vi "Loader RT Post-Build Action.vi"(5 "Files Generated by Build":path[](array[path]), 6 "Top Level/Always Included VIs":path[](array[path]), 7 "Destination Path":path, 8 "error in (no error)":errorcluster, 9 "Target Name":string, 10 "Build Specification Name":string, 11 "Project Path":path) -> (0 "error out":errorcluster)   [LabVIEW 2021, in "CIF Manager Build Actions.lvlib"]
uses:
  CIF Manager Build Actions.lvlib
  <vilib>/CIF Foundation/CIF Utilities/File/File_CIF_U.lvlib
  <vilib>/CIF Foundation/CIF Core/CIFUtilities/CIFConfigurationFile/CIF Configuration File.lvlib
  <vilib>/CIF Foundation/CIF Core/CIFUtilities/CIFConfigurationFile/typedef/Location Type.ctl
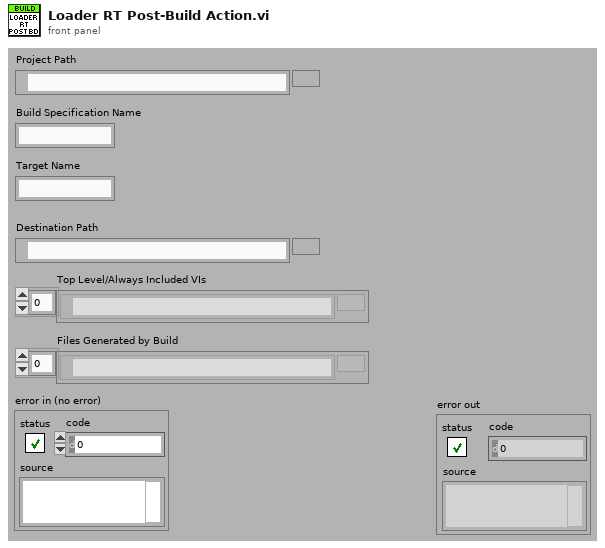
[diagram p1: front panel]
types:
  T1 = typedef "CIF Configuration File.lvlib/Location Type.ctl" = enum16{"Config File", "Manager", "Protos", "Plugins", "UI Plugins", "Logs", "Orchestrations", "Loaders"}
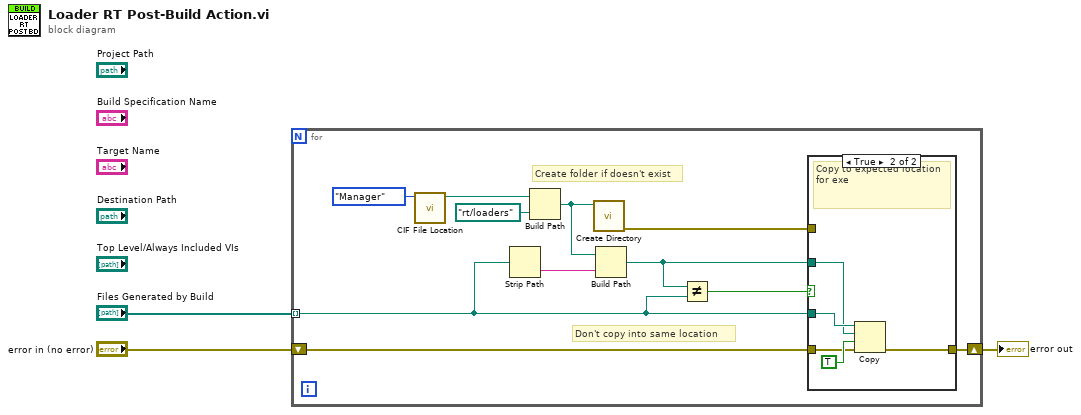
[diagram p0: block diagram]
diagram:
  n1 = for {
    tunnel: "Files Generated by Build" -> [w10] mode=indexing
    shift-right: [w14] -> w1
    shift-left: "error in (no error)" -> [w9]
    # "Create folder if doesn't exist"
    # "Don't copy into same location"
    n2 = call <vilib>:"CIF File Location.vi"("LocationType"=Location_Type."Manager") -> ("Location"=w6:path)  [unwired: 10 in]
    n3 = Strip Path(path=w10) -> (name=w11:string)  [unwired: 1 out]
    n4 = Build Path(base path=w6, name or relative path=path "rt/loaders") -> (appended path=w4:path)
    n5 = call <vilib>:"Create Directory.vi"("Path In"=w4) -> ("error out"=w12:errorcluster)  [unwired: 9 in, 1 out]
    n6 = Build Path(base path=w4, name or relative path=w11) -> (appended path=w13:path)
    n7 = Not Equal?(x=w13, y=w10) -> (x != y?=w8:bool)
    n8 = case shown="True" w8 {
      tunnel: w10 -> [_ w20]
      tunnel: w13 -> [_ w19]
      tunnel: w9 -> [w15 w17]
      tunnel: [w15 w16] -> w14
      tunnel: w12 -> [_ _]
      frame False {
        # "PPL not found, could provide error"
      }
      frame True {
        # "Copy to expected location for exe"
        n9 = Copy(8:w17, 9:TRUE ("overwrite (F)"), 10:w19, 11:w20) -> (0:w16:errorcluster)  [unwired: 1 in, 2 out]
      }
    }
  }
  "error out" <- w1
